vi "Receive Shortcut Menu Selection Event.vi"(8 "error in (no error)":errorcluster, 10 "ShortcutMenuSelectionMsg":refnum<class "ShortcutMenuSelectionMsg.lvclass">, 11 "Subroutine Dialog In":refnum<class "Subroutine Dialog.lvclass">) -> (0 "error out":errorcluster, 3 "Subroutine Dialog Out":refnum<class "Subroutine Dialog.lvclass">)   [LabVIEW 2017, in "Subroutine Dialog.lvclass"]
doc: "<License>\nCopyright © 2017 Composed Systems, LLC | All rights reserved\nwww.composed.io\n\nAuthor: Ethan Stern <ethan.stern@composed.io>\n\nThis software is provided \"AS IS\" WITHOUT WARRANTIES, either express or implied, AND IS FOR EDUCATIONAL PURPOSES ONLY.\n</License>"
uses:
  Subroutine Dialog.lvclass
  <vilib>/gpm_packages/@cs/mva-viewable/Source/ActorEvents/IEventAggregator Messages/ShortcutMenuSelectionMsg/ShortcutMenuSelectionMsg.lvclass
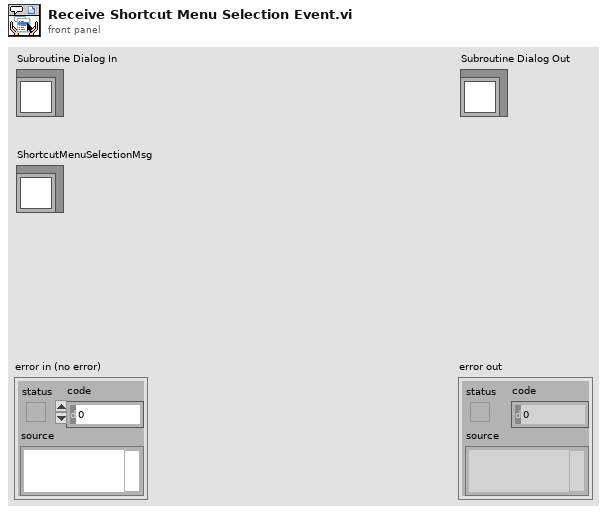
[diagram p1: front panel]
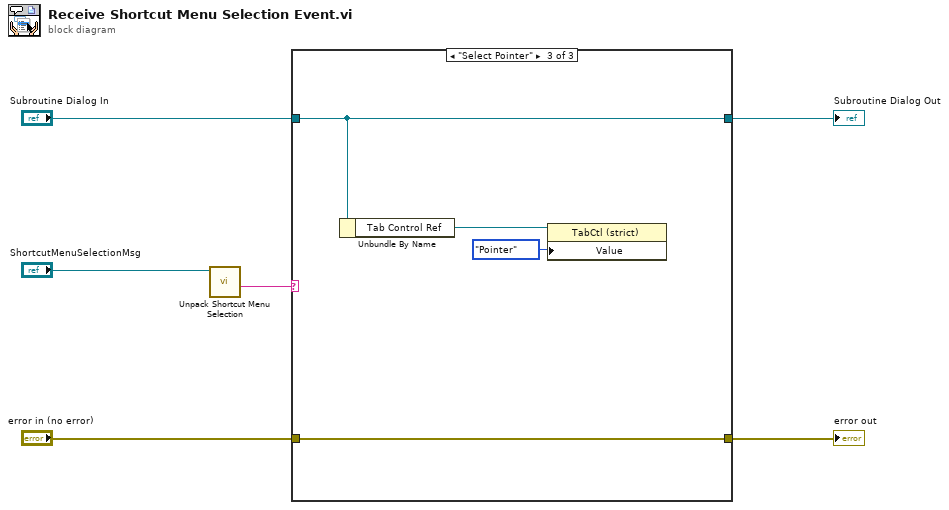
[diagram p0: block diagram]
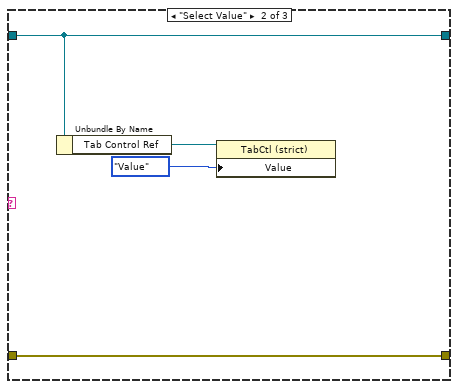
[diagram p3: hidden frame]
diagram:
  n1 = call <vilib>:"Unpack Shortcut Menu Selection.vi"("ShortcutMenuSelectionMsg"="ShortcutMenuSelectionMsg") -> ("Item Tag"=w3:string)  [unwired: 3 in, 7 out]
  n2 = case shown="\"Select Pointer\"" w3 {
    tunnel: "Subroutine Dialog In" -> [w8 w11 w13]
    tunnel: "error in (no error)" -> [w7 w12 w16]
    tunnel: [w8 w11 w13] -> w2
    tunnel: [w7 w12 w16] -> w1
    frame Default {
    }
    frame "Select Value" {
      n3 = Unbundle By Name(w11) -> ("Tab Control Ref"=w10:refnum<vi>)
      n4 = property class="TabCtl (strict)"(reference=w10, "Value"=enum32{"Value", "Pointer"}."Value") -> ()  [unwired: 1 in, 2 out]
    }
    frame "Select Pointer" {
      n5 = Unbundle By Name(w13) -> ("Tab Control Ref"=w15:refnum<vi>)
      n6 = property class="TabCtl (strict)"(reference=w15, "Value"=enum32{"Value", "Pointer"}."Pointer") -> ()  [unwired: 1 in, 2 out]
    }
  }
  "error out" <- w1
  "Subroutine Dialog Out" <- w2
